vi "SimpleExample_Ch1.vi"() -> ()   [LabVIEW 2016]
uses:
  <instrlib>/Rohde&Schwarz HMC 804x Power Supplies/Rohde&Schwarz HMC 804x Power Supplies.lvlib
panel:
  out "Screenshot":picture
  in  "CH1 Current":dbl=1.1
  in  "CH1 Voltage":dbl=3.0
  # "HMC804x simple example"
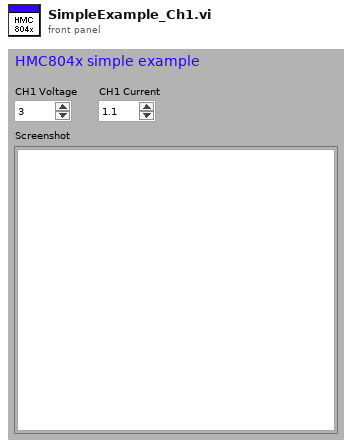
[diagram p1: front panel]
types:
  T1 = typedef "imagedata.ctl" = cluster{"image type":i32, "image depth":i32, "image":u8[], "mask":u8[], "colors":u32[], "Rectangle":cluster{"left":i16, "top":i16, "right":i16, "bottom":i16}}
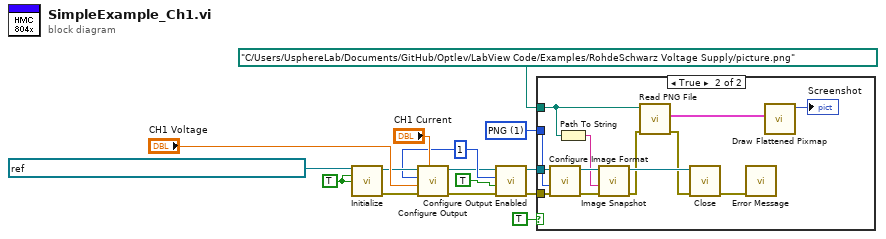
[diagram p0: block diagram]
diagram:
  w1 = 1 items=["BMP", "PNG"] ("Image Format (BMP)")
  w11 = TRUE ("ID Query (T: Check)")
  w12 = 1 ("Channel (1)")
  n1 = call <instrlib>:"Initialize.vi"("VISA resource name"=refnum<visa-resource-name> "USB0::0x0AAD::0x0197::5601.1414k02-100769::INSTR", "ID Query (T: Check)"=w11, "Reset (T: Reset)"=w11) -> ("VISA resource name out"=w13:refnum<visa-resource-name>, "error out"=w8:errorcluster)  [unwired: 11 in]
  n2 = call <instrlib>:"Configure Output.vi"("Current (0.0)"="CH1 Current", "error in (no error)"=w8, "Voltage (0.0)"="CH1 Voltage", "Channel (1)"=w12, "VISA resource name"=w13) -> ("error out"=w6:errorcluster, "VISA resource name out"=w7:refnum<visa-resource-name>)  [unwired: 5 in]
  n3 = call <instrlib>:"Configure Output Enabled.vi"("error in (no error)"=w6, "Enabled (Off)"=TRUE, "Channel (1)"=w12, "VISA resource name"=w7) -> ("error out"=w4:errorcluster, "VISA resource name out"=w5:refnum<visa-resource-name>)  [unwired: 6 in]
  n4 = case shown="True" TRUE {
    tunnel: path "C:/Users/UsphereLab/Documents/GitHub/Optlev/LabView Code/Examples/RohdeSchwarz Voltage Supply/picture.png" ("path to BMP file") -> [_ w23]
    tunnel: w5 -> [_ w18]
    tunnel: w4 -> [_ w17]
    tunnel: w1 -> [_ w16]
    frame False {
    }
    frame True {
      n5 = call <instrlib>:"Configure Image Format.vi"("error in (no error)"=w17, "Image Format (BMP)"=w16, "VISA resource name"=w18) -> ("error out"=w22:errorcluster, "VISA resource name out"=w25:refnum<visa-resource-name>)  [unwired: 7 in]
      n6 = Path To String(path=w23) -> (string=w24:string)
      n7 = call <instrlib>:"Image Snapshot.vi"("error in (no error)"=w22, "Destination (\"\")"=w24, "VISA resource name"=w25) -> ("error out"=w21:errorcluster, "VISA resource name out"=w26:refnum<visa-resource-name>)  [unwired: 7 in]
      n8 = call <vilib>:"Read PNG File.vi"("error in (no error)"=w21, "path to PNG file"=w23) -> ("error out"=w20:errorcluster, "image data"=w28:T1)  [unwired: 7 in, 1 out]
      n9 = call <instrlib>:"Close.vi"("error in (no error)"=w20, "VISA resource name"=w26) -> ("error out"=w19:errorcluster)  [unwired: 9 in]
      n10 = call <instrlib>:"Error Message.vi"("error in (no error)"=w19) -> ()  [unwired: 10 in, 5 out]
      n11 = call <vilib>:"Draw Flattened Pixmap.vi"("image data"=w28) -> ("new picture"=→"Screenshot":picture)  [unwired: 8 in]
    }
  }
